vi "ALTS-2015 Check for UUT Clamped and then Start.vi"(8 "error in":errorcluster, 11 "Station Cluster":T1) -> (0 "error out":errorcluster)   [LabVIEW 2013]
doc: "Copyright © 2005, Soliton Technologies.\nAll rights reserved."
uses:
  Controls/ALTS-2015 Station Cluster.ctl
  Controls/ALTS-2015 Status Message Options.ctl
  Controls/ALTS-2015 LV2GBL Station Info Options.ctl
  Controls/ALTS-2015 Ring Indicator Enum.ctl
  Controls/ALTS-2015 Status Ring Indicator.ctl
  Controls/ALTS-2015 DO Start Stop Options.ctl
  Controls/ALTS-2015 Digital Output Options.ctl
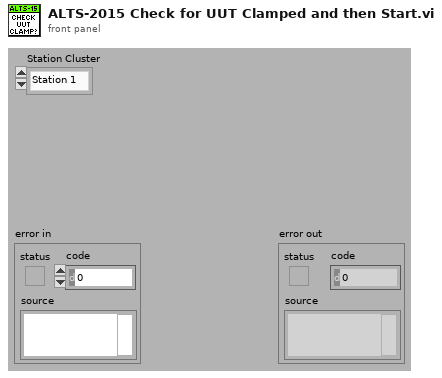
[diagram p1: front panel]
types:
  T1 = typedef "ALTS-2015 Station Cluster.ctl" = enum16{"Station 1", "Station 2", "Station 3", "Station 4"}
  T2 = typedef "ALTS-2015 Status Message Options.ctl" = enum16{"Initializing...", "Enter User Login...", "Enter Work Order Number...", "Enter Serial Number...", "Valid Serial Number...", "Invalid Serial Number...", "Start Tag Received...", "Stop Tag Received...", "UUT Clamped...", "UUT not Clamped...", "Test Running...", "Test Complete...", "Writing Result to DB...", "DB Entry Pressed...", "Clearing Serial Number...", "Idle...", "Exiting..."}
  T3 = typedef "ALTS-2015 LV2GBL Station Info Options.ctl" = enum16{"Init", "Read", "Read All", "Write Sensor ID", "Write  WO & SN", "Write Test Data", "Write Station Status", "Clear All", "Clear Test Result"}
  T4 = typedef "ALTS-2015 Status Ring Indicator.ctl" = u16
  T5 = typedef "ALTS-2015 Ring Indicator Enum.ctl" = enum16{"Idle", "Test Running", "Unit Clamped", "Unit not Clamped", "Pass", "Fail"}
  T6 = typedef "ALTS-2015 Digital Output Options.ctl" = enum16{"Idle", "Test Running", "Pass", "Fail"}
  T7 = typedef "ALTS-2015 DO Start Stop Options.ctl" = enum16{"Start Test", "Stop Test"}
  T8 = typedef "ALTS-2015 Station Details.ctl" = cluster{"Station Number":string, "Work Order Number":string, "Sensor Name":string, "Pressure (PSI)":string, "Flow (SCCM)":string, "Test Time ":string, "Test Result":string, "Serial Number":string, "Station Status":T4, "Station Occupied?":bool, "Rerun Count":i32}
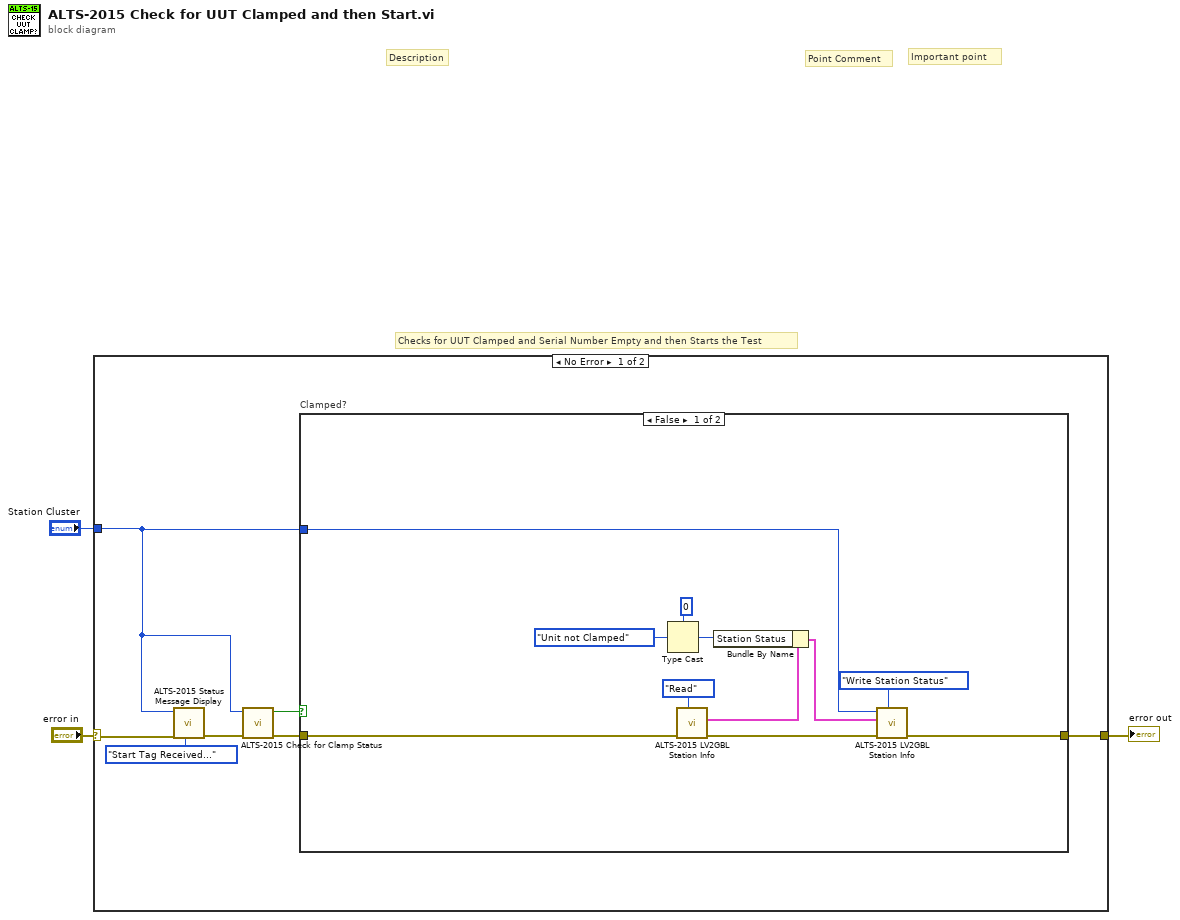
[diagram p0: block diagram]
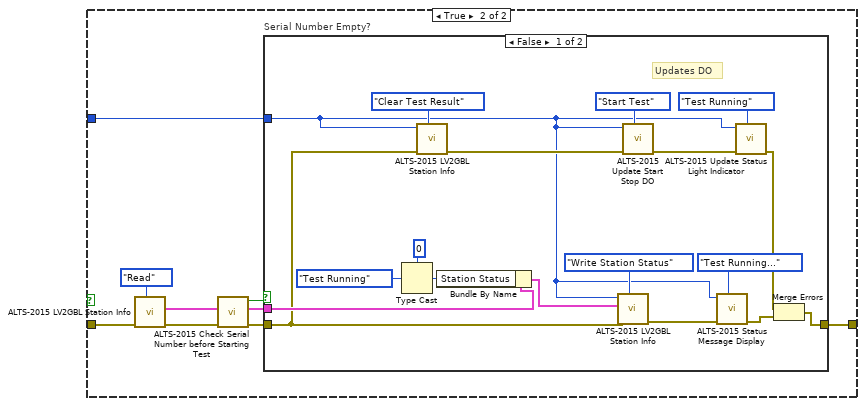
[diagram p2: hidden frame]
diagram:
  # "Checks for UUT Clamped and Serial Number Empty and then Starts the Test"
  # "Point Comment"
  # "Important point"
  # "Description"
  n1 = case shown="No Error" "error in" {
    selector: "error in" -> [w6 w50]
    tunnel: [w5 w50] -> w2
    tunnel: "Station Cluster" -> [w4 _]
    frame No Error {
      n2 = call "ALTS-2015 Status Message Display.vi"("Status Message Options"=ALTS-2015_Status_Message_Options."Start Tag Received...", "error in (no error)"=w6, "Station Enum"=w4) -> ("error out"=w7:errorcluster)  [unwired: 7 in, 1 out]
      n3 = call "ALTS-2015 Check for Clamp Status .vi"("error in (no error)"=w7, "Station Cluster"=w4) -> ("error out"=w10:errorcluster, "Clamp?"=w9:bool)  [unwired: 8 in]
      n4 = case "Clamped?" shown="False" w9 {
        tunnel: w10 -> [w13 w28]
        tunnel: [w18 w30] -> w5
        tunnel: w4 -> [w19 w27]
        frame False {
          n5 = Type Cast(type=T4 0 ("Station Status"), x=ALTS-2015_Ring_Indicator_Enum."Unit not Clamped" ("Ring Indicator Options")) -> (*(type *) &x=w15:T4)
          n6 = call "ALTS-2015 LV2GBL Station Info.vi"("Options"=ALTS-2015_LV2GBL_Station_Info_Options."Read", "error in"=w13) -> ("error out"=w12:errorcluster, "Station Details"=w11:T8)  [unwired: 7 in, 1 out]
          n7 = Bundle By Name(cluster=w11, "Station Status"=w15) -> (w20:T8)
          n8 = call "ALTS-2015 LV2GBL Station Info.vi"("Options"=ALTS-2015_LV2GBL_Station_Info_Options."Write Station Status", "error in"=w12, "Station"=w20, "Station Cluster"=w19) -> ("error out"=w18:errorcluster)  [unwired: 5 in, 2 out]
        }
        frame True {
          n9 = call "ALTS-2015 LV2GBL Station Info.vi"("Options"=ALTS-2015_LV2GBL_Station_Info_Options."Read", "error in"=w28) -> ("error out"=w24:errorcluster, "Station Details"=w26:T8)  [unwired: 7 in, 1 out]
          n10 = call "ALTS-2015 Check Serial Number before Starting Test.vi"("error in (no error)"=w24, "Station Details"=w26) -> ("error out"=w23:errorcluster, "Station Details Out"=w25:T8, "SN Empty?"=w22:bool)  [unwired: 7 in]
          n11 = case "Serial Number Empty?" shown="False" w22 {
            tunnel: [w46 w49] -> w30
            tunnel: w27 -> [w34 _]
            tunnel: w25 -> [w40 _]
            tunnel: w23 -> [w36 w49]
            frame False {
              # "Updates DO"
              n12 = Type Cast(type=T4 0 ("Station Status"), x=ALTS-2015_Ring_Indicator_Enum."Test Running" ("Ring Indicator Options")) -> (*(type *) &x=w31:T4)
              n13 = call "ALTS-2015 LV2GBL Station Info.vi"("Options"=ALTS-2015_LV2GBL_Station_Info_Options."Clear Test Result", "error in"=w36, "Station Cluster"=w34) -> ("error out"=w35:errorcluster)  [unwired: 6 in, 2 out]
              n14 = Bundle By Name(cluster=w40, "Station Status"=w31) -> (w43:T8)
              n15 = call "ALTS-2015 LV2GBL Station Info.vi"("Options"=ALTS-2015_LV2GBL_Station_Info_Options."Write Station Status", "error in"=w36, "Station"=w43, "Station Cluster"=w34) -> ("error out"=w44:errorcluster)  [unwired: 5 in, 2 out]
              n16 = call "ALTS-2015 Update Start Stop DO.vi"("DO Options"=ALTS-2015_DO_Start_Stop_Options."Start Test", "error in"=w35, "Station Cluster"=w34) -> ("error out"=w48:errorcluster)  [unwired: 8 in]
              n17 = call "ALTS-2015 Status Message Display.vi"("Status Message Options"=ALTS-2015_Status_Message_Options."Test Running...", "error in (no error)"=w44, "Station Enum"=w34) -> ("error out"=w38:errorcluster)  [unwired: 7 in, 1 out]
              n18 = call "ALTS-2015 Update Status Light Indicator.vi"("DO Options"=ALTS-2015_Digital_Output_Options."Test Running", "error in"=w48, "Station Cluster"=w34) -> ("error out"=w39:errorcluster)  [unwired: 8 in]
              n19 = Merge Errors(w39, w38) -> (w46:errorcluster)
            }
            frame True {
            }
          }
        }
      }
    }
    frame Error {
    }
  }
  "error out" <- w2
